vi "CMN_GetCommFile.vi"(8 "error in (no error)":errorcluster, 10 "path in":path) -> (0 "error out":errorcluster, 2 "path out":path)   [LabVIEW 2016]
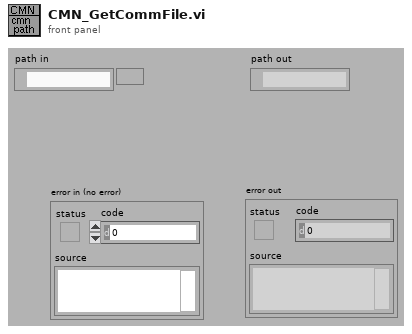
[diagram p1: front panel]
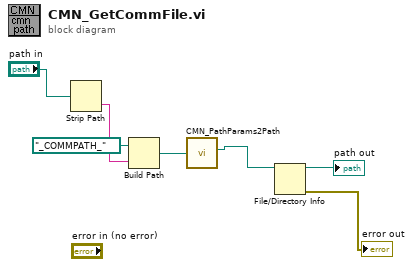
[diagram p0: block diagram]
diagram:
  n1 = Strip Path(path="path in") -> (name=w6:string)  [unwired: 1 out]
  n2 = Build Path(base path=path "_COMMPATH_", name or relative path=w6) -> (appended path=w4:path)
  n3 = call "CMN_PathParams2Path.vi"("Path In"=w4) -> ("Path out"=w3:path)  [unwired: 2 in, 8 out]
  n4 = File/Directory Info(path=w3) -> (path out=→"path out":path, error out=→"error out":errorcluster)  [unwired: 1 in, 5 out]
